vi "Set All Parameters.vi"(8 "error in (no error)":errorcluster, 10 "Parameters":T1={"Type"=enum."Mouse Move", "X"=0, "Y"=0, "Delay"=0, "Key"=65, "Repeat"=0, "RClick?"=FALSE, "App/Window Name"="", "Notes"="", "Assertion Type"=enum."Control Position", "Control Name"="", "Stop on Fail?"=FALSE, "Disabled"=enum."Enabled", "Visible"=enum."Visible", "Left"=0, "Top"=0, "Width"=0, "Height"=0, "Expected Image"={"image type"=0, "image depth"=0, "image"=[], "mask"=[], "colors"=[], "Rectangle"={"left"=0, "top"=0, "right"=0, "bottom"=0}}}, 11 "Window Action in":refnum<class "Window Action.lvclass">) -> (0 "error out":errorcluster, 3 "Window Action out":refnum<class "Window Action.lvclass">)   [LabVIEW 2020, in "MacroAssert.lvlib" / "Window Action.lvclass"]
uses:
  Step/Step.lvclass
  Window Action.lvclass
  Window Action.lvclass/Window Action.ctl
  Action Step/Action Step.lvclass
  CTLs/Step Type V3.ctl
  MacroAssert.lvlib
  CTLs/Assertion Type.ctl
  <vilib>/picture/picture.llb/imagedata.ctl
  CTLs/Step V3.ctl
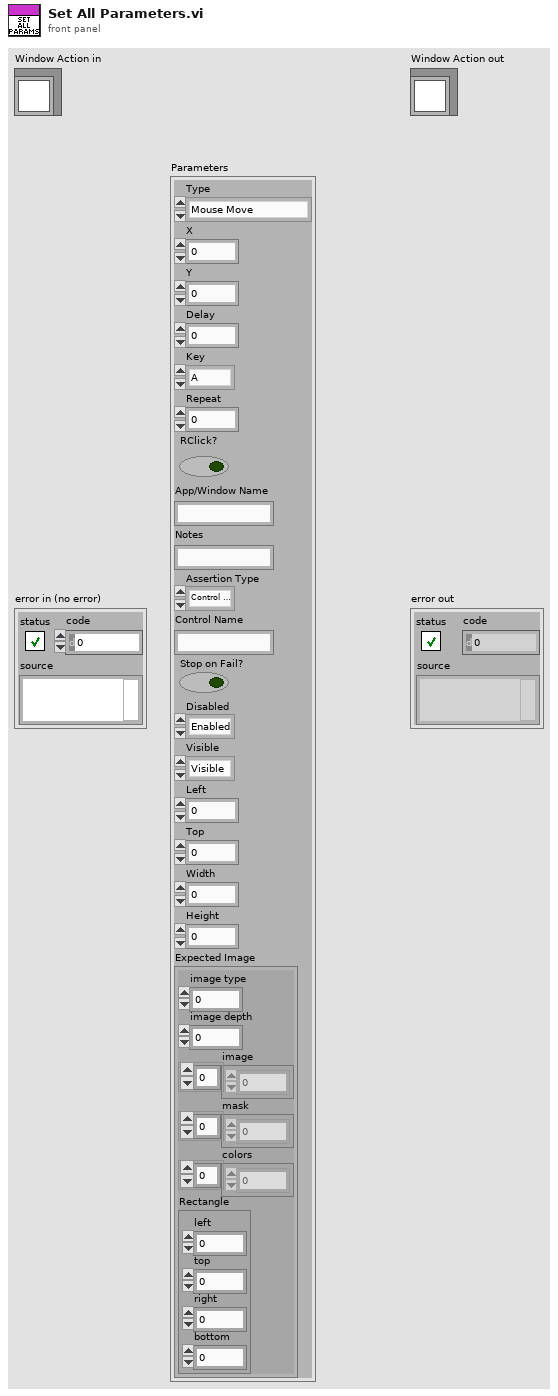
[diagram p1: front panel]
types:
  T1 = typedef "MacroAssert.lvlib/Step V3.ctl" = cluster{"Type":T2, "X":i32, "Y":i32, "Delay":i32, "Key":u8, "Repeat":i32, "RClick?":bool, "App/Window Name":string, "Notes":string, "Assertion Type":T3, "Control Name":string, "Stop on Fail?":bool, "Disabled":enum8{"Enabled", "Disabled", "Disabled and Grayed Out"}, "Visible":enum16{"Visible", "Not Visible"}, "Left":i16, "Top":i16, "Width":i16, "Height":i16, "Expected Image":T4}
  T2 = typedef "MacroAssert.lvlib/Step Type V3.ctl" = enum16{"Mouse Move", "Mouse Click", "Key Press", "Wait", "Mouse Down", "Mouse Up", "Key Down", "Key Up", "Maximize Window", "Restore Window", "Minimize Window", "Close Window", "Bring Window to Front", "Send Window to Back", "Assertion: Ctl Visible", "Assertion: Ctl Disabled", "Assertion: Ctl Image"}
  T3 = typedef "MacroAssert.lvlib/Assertion Type.ctl" = enum16{"Control Position", "Control Visible", "Control Disabled", "Control Image"}
  T4 = typedef "imagedata.ctl" = cluster{"image type":i32, "image depth":i32, "image":u8[], "mask":u8[], "colors":u32[], "Rectangle":cluster{"left":i16, "top":i16, "right":i16, "bottom":i16}}
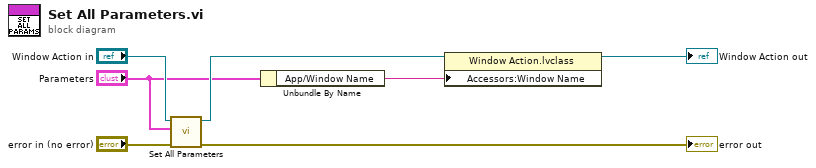
[diagram p0: block diagram]
diagram:
  n1 = call-parent "Set All Parameters.vi"("error in (no error)"="error in (no error)", "Parameters"="Parameters", "Action Step in"="Window Action in") -> ("error out"=→"error out":errorcluster, "Action Step out"=w3:refnum<class "Window Action.lvclass">)  [unwired: 7 in]
  n2 = Unbundle By Name("Parameters") -> ("App/Window Name"=w4:string)
  n3 = property class="Window Action.lvclass"(reference=w3, "Accessors:Window Name"=w4) -> (reference out=→"Window Action out":refnum<class "Window Action.lvclass">)  [unwired: 1 in, 1 out]
